vi "Execute Buffer Reset.vi"(8 "error in":errorcluster, 11 "CPC in":refnum<class "CPC.lvclass">) -> (0 "error out":errorcluster, 2 "CMD Good":bool, 3 "CPC out":refnum<class "CPC.lvclass">)   [LabVIEW 2013, in "CPC.lvclass"]
uses:
  CPC.lvclass
  CPC.lvclass/CPC.ctl
  Reusable/Session APIs/Serial/Public/Get Data/Get String.vi
  Reusable/Session APIs/Serial/Serial Session.lvclass
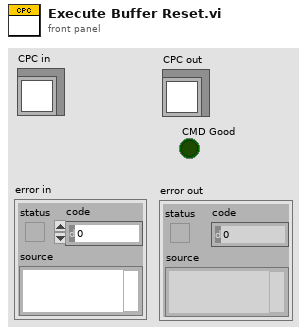
[diagram p1: front panel]
types:
  T1 = typedef "Serial Session.lvclass/Session Handle.ctl" = refnum<data-value>
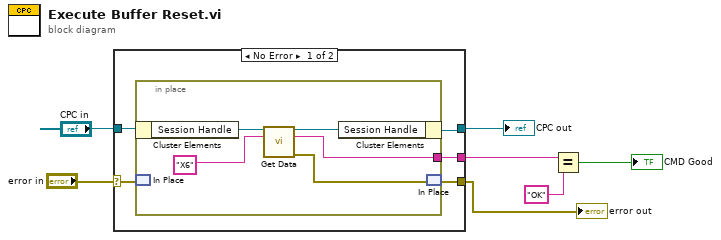
[diagram p0: block diagram]
diagram:
  n1 = case shown="No Error" "error in" {
    selector: "error in" -> [w11 w19]
    tunnel: "CPC in" -> [w12 w18]
    tunnel: [w9 w19] -> w3
    tunnel: [w10 w18] -> w1
    tunnel: [w8 _] -> w6
    frame No Error {
      n2 = in-place {
        in-place-border: [w14] -> w8
        n3 = in-place-cluster #1(w12) -> ("Session Handle"=w17:T1)
        n4 = in-place-match #2(w11) -> ()  [unwired: 1 out]
        n5 = call-poly "Get Data.vi"("Session Handle in"=w17, "CMD"="X6" ("string")) -> ("Session Handle out"=w16:T1, "DataOut"=w14:string, "error out"=w15:errorcluster)  [unwired: 11 in]
        n6 = in-place-cluster #1("Session Handle"=w16) -> (w10:refnum<class "CPC.lvclass">)
        n7 = in-place-match #2(w15) -> (w9:errorcluster)
      }
    }
    frame Error {
    }
  }
  "error out" <- w3
  "CPC out" <- w1
  n8 = Equal?(x=w6, y="OK") -> (x = y?=→"CMD Good":bool)
